vi "Loop Get ShiftRegister Input Output Assignements.vi"(10 "Inside Terms[] offset 2":i32, 11 "RightShiftRegister[]":refnum<vi>[](array[refnum])) -> (1 "init values":string, 2 "output assignements":string, 3 "input assignements":string)   [LabVIEW 2014]
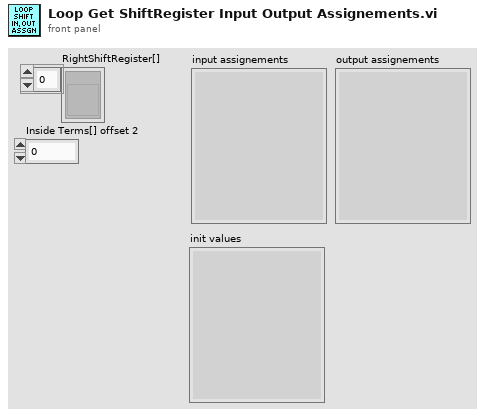
[diagram p1: front panel]
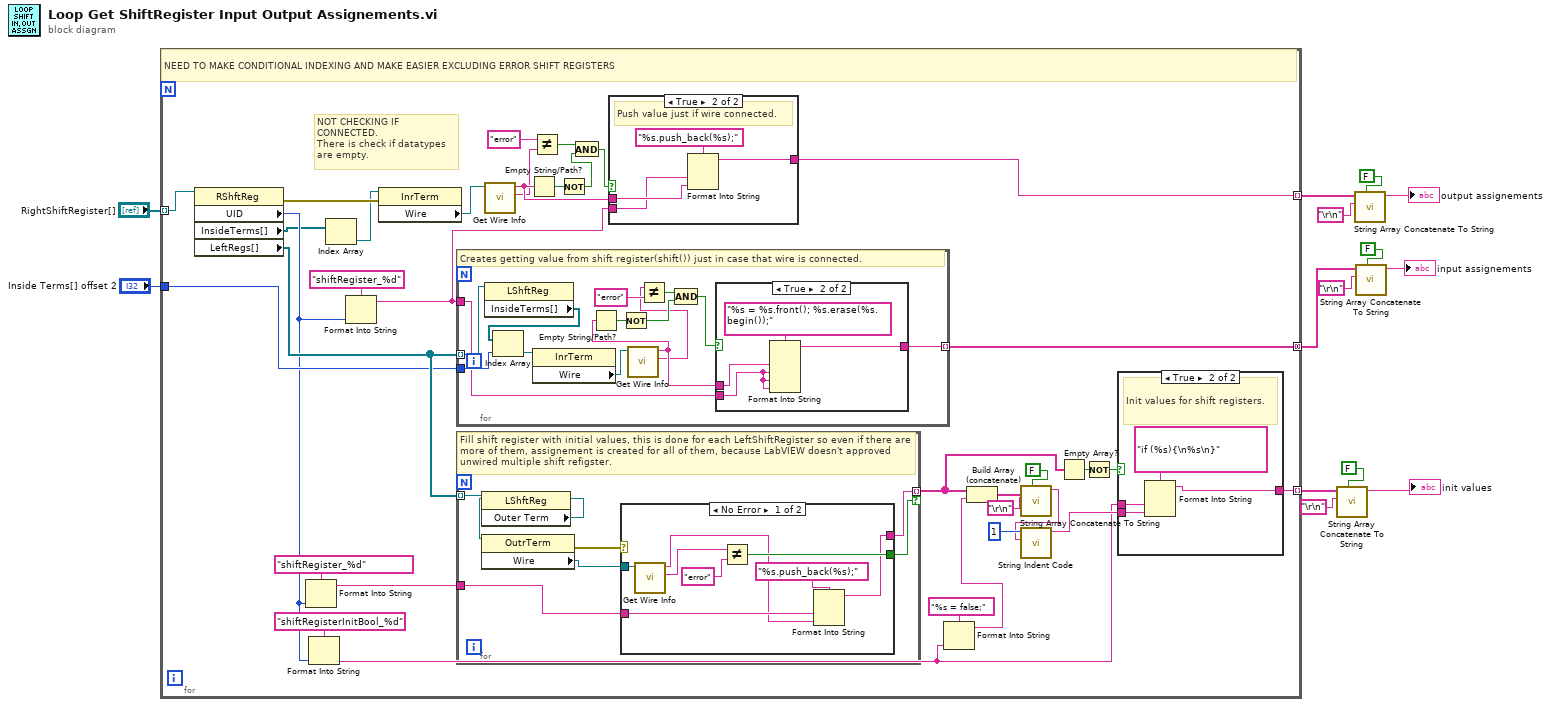
[diagram p0: block diagram]
diagram:
  n1 = for {
    tunnel: "RightShiftRegister[]" -> [w48] mode=indexing
    tunnel: "Inside Terms[] offset 2" -> [w31]
    tunnel: [w45] -> w6 mode=concatenating
    tunnel: [w41] -> w7 mode=indexing
    tunnel: [w30] -> w1 mode=indexing
    # "NOT CHECKING IF CONNECTED.\nThere is check if datatypes are empty."
    # "NEED TO MAKE CONDITIONAL INDEXING AND MAKE EASIER EXCLUDING ERROR SHIFT REGISTERS"
    n2 = property class="RShftReg"(reference=w48) -> (error out=w49:errorcluster, "UID"=w22:i32, "InsideTerms[]"=w16:refnum<vi>[], "LeftRegs[]"=w35:refnum<vi>[])  [unwired: 1 in, 1 out]
    n3 = Format Into String(format string="shiftRegister_%d", w22) -> (resulting string=w20:string)  [unwired: 2 in, 1 out]
    n4 = Format Into String(format string="shiftRegisterInitBool_%d", w22) -> (resulting string=w18:string)  [unwired: 2 in, 1 out]
    n5 = Index Array(array=w16) -> (element=w15:refnum<vi>)  [unwired: 1 in]
    n6 = Format Into String(format string="shiftRegister_%d", w22) -> (resulting string=w43:string)  [unwired: 2 in, 1 out]
    n7 = property class="InrTerm"(reference=w15, error in=w49) -> ("Wire"=w47:refnum<vi>)  [unwired: 2 out]
    n8 = for {
      tunnel: w31 -> [w83]
      tunnel: w35 -> [w80] mode=indexing
      tunnel: w43 -> [w76]
      tunnel: [w74] -> w45 mode=indexing
      # "Creates getting value from shift register(shift()) just in case that wire is connected."
      n9 = property class="LShftReg"(reference=w80) -> ("InsideTerms[]"=w79:refnum<vi>[])  [unwired: 1 in, 2 out]
      n10 = Index Array(array=w79, index=w83) -> (element=w78:refnum<vi>)
      n11 = property class="InrTerm"(reference=w78) -> ("Wire"=w86:refnum<vi>)  [unwired: 1 in, 2 out]
      n12 = call "Get Wire Info.vi"("Wire"=w86) -> ("wire datatype"=w73:string, "wire label"=w75:string)  [unwired: 9 in]
      n13 = Empty String/Path?(string/path=w75) -> (empty?=w82:bool)
      n14 = Not(x=w82) -> (.not. x?=w81:bool)
      n15 = Not Equal?(x=w73, y="error") -> (x != y?=w85:bool)
      n16 = Compound Arithmetic op=AND(w85, w81) -> (w77:bool)
      n17 = case shown="True" w77 {
        tunnel: w76 -> [_ w87]
        tunnel: w75 -> [_ w89]
        tunnel: [_ w88] -> w74
        frame False {
        }
        frame True {
          n18 = Format Into String(format string="%s = %s.front(); %s.erase(%s.begin());", w89, w87, w87, w87) -> (resulting string=w88:string)  [unwired: 2 in, 1 out]
        }
      }
    }
    n19 = for {
      tunnel: w35 -> [w60] mode=indexing
      tunnel: [w56] -> w23 mode=indexing if=w55
      tunnel: w20 -> [w54]
      # "Fill shift register with initial values, this is done for each LeftShiftRegister so even if there are more of them, assignement is created for all of them, because LabVIEW doesn't approved unwired multiple shift refigster."
      n20 = property class="LShftReg"(reference=w60) -> ("Outer Term"=w59:refnum<vi>)  [unwired: 1 in, 2 out]
      n21 = property class="OutrTerm"(reference=w59) -> (error out=w57:errorcluster, "Wire"=w58:refnum<vi>)  [unwired: 1 in, 1 out]
      n22 = case shown="No Error" w57 {
        tunnel: w58 -> [w68 _]
        tunnel: [w66 _] -> w55
        tunnel: [w61 _] -> w56
        tunnel: w54 -> [w63 _]
        frame No Error {
          n23 = call "Get Wire Info.vi"("Wire"=w68) -> ("wire datatype"=w65:string, "wire label"=w62:string)  [unwired: 9 in]
          n24 = Not Equal?(x=w65, y="error") -> (x != y?=w66:bool)
          n25 = Format Into String(format string="%s.push_back(%s);", w63, w62) -> (resulting string=w61:string)  [unwired: 2 in, 1 out]
        }
        frame Error {
        }
      }
    }
    n26 = call "Get Wire Info.vi"("Wire"=w47) -> ("wire datatype"=w37:string, "wire label"=w42:string)  [unwired: 9 in]
    n27 = Empty String/Path?(string/path=w42) -> (empty?=w44:bool)
    n28 = Not Equal?(x="error" ("y"), y=w37) -> (x != y?=w39:bool)
    n29 = Not(x=w44) -> (.not. x?=w40:bool)
    n30 = And(x=w39, y=w40) -> (x .and. y?=w36:bool)
    n31 = case shown="True" w36 {
      tunnel: w43 -> [_ w69]
      tunnel: w42 -> [_ w70]
      tunnel: [_ w71] -> w41
      frame False {
      }
      frame True {
        # "Push value just if wire connected."
        n32 = Format Into String(format string="%s.push_back(%s);", w69, w70) -> (resulting string=w71:string)  [unwired: 2 in, 1 out]
      }
    }
    n33 = Format Into String(format string="%s = false;", w18) -> (resulting string=w17:string)  [unwired: 2 in, 1 out]
    n34 = Build Array (concatenate)(w23, w17) -> (w28:string[])
    n35 = call "String Array Concatenate To String.vi"("insert last delimiter?"=FALSE, "Delimiter char"="\r\n", "Array String In"=w28) -> ("String"=w26:string)  [unwired: 8 in]
    n36 = call "String Indent Code.vi"("complete code"=w26, "actual nested level"=1) -> ("indented code"=w25:string)  [unwired: 9 in]
    n37 = Empty Array?(array=w23) -> (empty?=w24:bool)
    n38 = Not(x=w24) -> (.not. x?=w29:bool)
    n39 = case shown="True" w29 {
      tunnel: w18 -> [_ w52]
      tunnel: w25 -> [_ w51]
      tunnel: [_ w50] -> w30
      frame False {
        # "Remove error shift registers."
      }
      frame True {
        # "Init values for shift registers."
        n40 = Format Into String(format string="if (%s){\n%s\n}", w52, w51) -> (resulting string=w50:string)  [unwired: 2 in, 1 out]
      }
    }
  }
  n41 = call "String Array Concatenate To String.vi"("insert last delimiter?"=FALSE, "Delimiter char"="\r\n", "Array String In"=w1) -> ("String"=→"init values":string)  [unwired: 8 in]
  n42 = call "String Array Concatenate To String.vi"("insert last delimiter?"=FALSE, "Delimiter char"="\r\n", "Array String In"=w7) -> ("String"=→"output assignements":string)  [unwired: 8 in]
  n43 = call "String Array Concatenate To String.vi"("insert last delimiter?"=FALSE, "Delimiter char"="\r\n", "Array String In"=w6) -> ("String"=→"input assignements":string)  [unwired: 8 in]
